vi "Call Keep IE in Memory.vi"   [LabVIEW 2020]
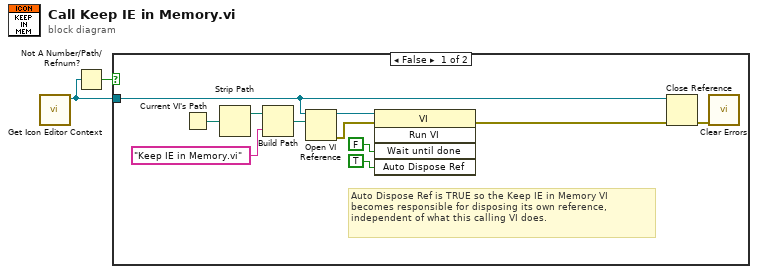
[diagram p0: block diagram]
diagram:
  n1 = call "Get Icon Editor Context.vi"() -> ("icon editor context"=w2:refnum<vi>)  [unwired: 11 in]
  n2 = Not A Number/Path/Refnum?(number/path/refnum=w2) -> (NaN/Path/Refnum?=w1:bool)
  n3 = case shown="False" w1 {
    tunnel: w2 -> [w3 _]
    frame False {
      # "Auto Dispose Ref is TRUE so the Keep IE in Memory VI becomes responsible for disposing its own reference, independent of what this calling VI does."
      n4 = Current VI's Path() -> (path=w11:path)
      n5 = Strip Path(path=w11) -> (stripped path=w10:path)  [unwired: 1 out]
      n6 = Build Path(base path=w10, name or relative path="Keep IE in Memory.vi") -> (appended path=w8:path)
      n7 = Open VI Reference(application reference (local)=w3, vi path=w8) -> (vi reference=w7:refnum<vi>, error out=w6:errorcluster)  [unwired: 1 in, 3 out]
      n8 = invoke class="VI" method="Run VI"(reference=w7, error in=w6, "Wait until done"=FALSE ("Wait Until Done"), "Auto Dispose Ref"=TRUE ("Auto Dispose Reference")) -> (error out=w5:errorcluster)  [unwired: 1 in, 4 out]
      n9 = Close Reference(reference=w3, error in (no error)=w5) -> (error out=w4:errorcluster)
      n10 = call <vilib>:"Clear Errors.vi"("error in (no error)"=w4) -> ()  [unwired: 5 in, 2 out]
    }
    frame True {
    }
  }
